vi "file.valid.vi"(8 "error in":errorcluster, 11 "midi-file in":refnum<class "midi-file.lvclass">) -> (0 "error out":errorcluster, 3 "midi-file out":refnum<class "midi-file.lvclass">)   [LabVIEW 2020, in "midi-file.lvclass"]
uses:
  midi-file.lvclass
  midi-file.lvclass/midi-file.ctl
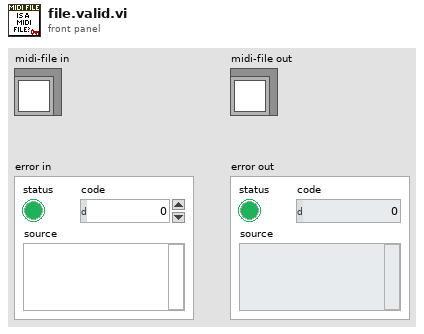
[diagram p1: front panel]
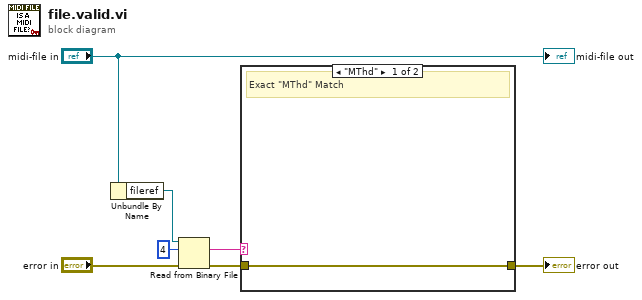
[diagram p0: block diagram]
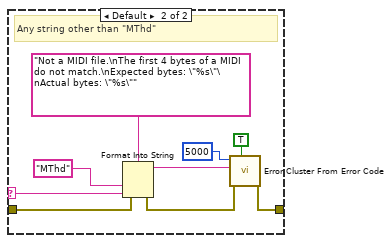
[diagram p2: hidden frame]
diagram:
  n1 = Unbundle By Name("midi-file in") -> ("fileref"=w7:refnum<file>)
  n2 = Read from Binary File(8:"error in", 10:4 ("count (1)"), 11:w7) -> (0:w3:errorcluster, 2:w4:string)  [unwired: 3 in, 2 out]
  n3 = case shown="\"MThd\"" w4 {
    selector: w4 -> [_ w12]
    tunnel: w3 -> [w8 w10]
    tunnel: [w8 w9] -> w2
    frame "MThd" {
      # "Exact \"MThd\" Match"
    }
    frame Default {
      # "Any string other than \"MThd\""
      n4 = Format Into String(format string="Not a MIDI file.\nThe first 4 bytes of a MIDI do not match.\nExpected bytes: \"%s\"\nActual bytes: \"%s\"" ("error message (\"\")"), error in=w10, "MThd" ("y"), w12) -> (resulting string=w14:string, error out=w11:errorcluster)  [unwired: 1 in]
      n5 = call <vilib>:"Error Cluster From Error Code.vi"("show call chain? (False)"=TRUE, "error in (no error)"=w11, "error message (\"\")"=w14, "error code (0)"=5000) -> ("error out"=w9:errorcluster)  [unwired: 5 in]
    }
  }
  "error out" <- w2
  "midi-file out" <- "midi-file in"
